vi "AerotechGetState.vi"(0 "error in (no error)":errorcluster) -> (3 "error out":errorcluster, 5 "State":T1)   [LabVIEW 2009]
uses:
  Controls/AerotechState.ctl
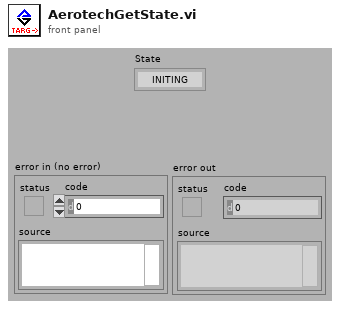
[diagram p1: front panel]
types:
  T1 = typedef "AerotechState.ctl" = enum16{"INITING", "IDLING", "SLEWING", "TRACKING", "MOVING", "HOMING", "STOPPING"}
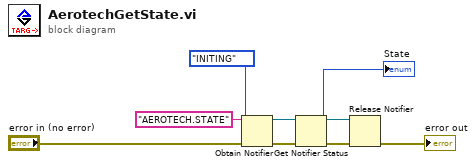
[diagram p0: block diagram]
diagram:
  n1 = Obtain Notifier(name (unnamed)="AEROTECH.STATE", notification data type=AerotechState."INITING" ("AEROTECH.ACTUAL"), error in (no error)="error in (no error)") -> (notifier out=w8:refnum<notifier>, error out=w3:errorcluster)  [unwired: 1 in, 1 out]
  n2 = Get Notifier Status(notifier=w8, error in (no error)=w3) -> (notifier out=w6:refnum<notifier>, current notification=→"State":T1, error out=w7:errorcluster)  [unwired: 2 out]
  n3 = Release Notifier(notifier=w6, error in (no error)=w7) -> (error out=→"error out":errorcluster)  [unwired: 1 in, 2 out]
